vi "Can Expand.vi"(11 "State":T1) -> (3 "Can Expand?":bool)   [LabVIEW 2020, in "Parallel Diagram Block.xnode"]
uses:
  Parallel Diagram Block.xnode
  Parallel Block/Value Type.ctl
  Parallel Block/Parallel Block.lvlib
  Parallel Block/Type Descriptor.ctl
  <vilib>/picture/picture.llb/imagedata.ctl
  Parallel Block/Direction.ctl
  Parallel Block/IO Selection.ctl
  State.ctl
  Parallel Block/Terminal Mode.ctl
  Parallel Block/Terminal Type.ctl
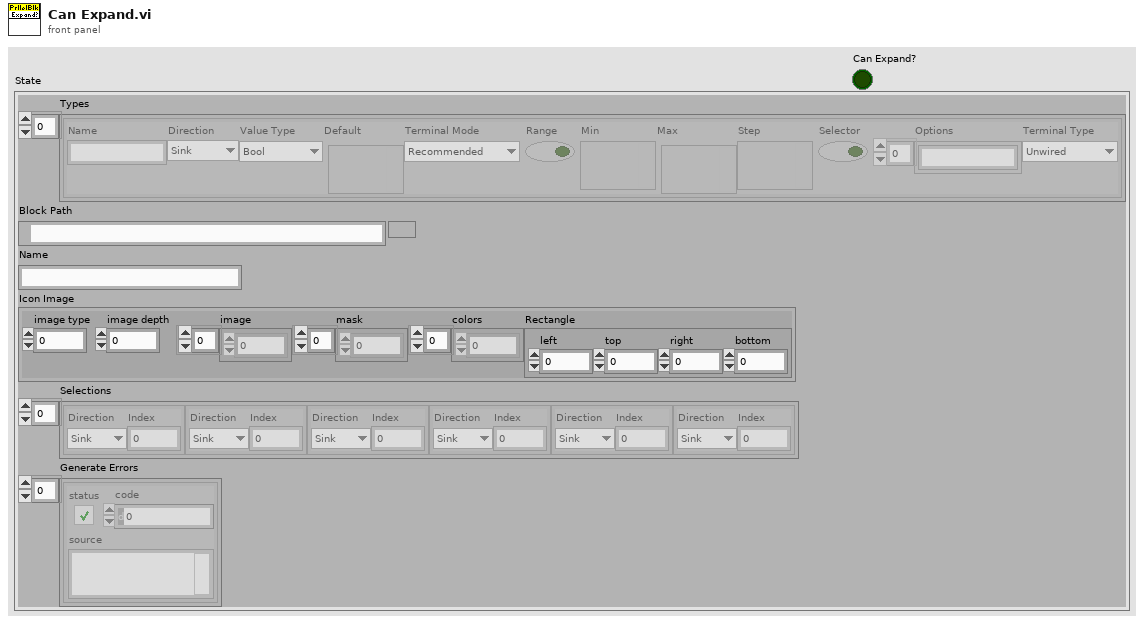
[diagram p1: front panel]
types:
  T1 = typedef "Parallel Diagram Block.xnode/State.ctl" = cluster{"Types":T2[], "Block Path":path, "Name":string, "Icon Image":T7, "Selections":T8[], "Generate Errors":errorcluster[]}
  T2 = typedef "Parallel Block.lvlib/Type Descriptor.ctl" = cluster{"Name":string, "Direction":T3, "Value Type":T4, "Default":variant, "Terminal Mode":T5, "Range":bool, "Min":variant, "Max":variant, "Step":variant, "Selector":bool, "Options":string[], "Terminal Type":T6}
  T3 = typedef "Parallel Block.lvlib/Direction.ctl" = enum16{"Sink", "Source"}
  T4 = typedef "Parallel Block.lvlib/Value Type.ctl" = enum16{"Unknown", "Bool", "U8", "U16", "U32", "U64", "I8", "I16", "I32", "I64", "SGL", "DBL", "CSG", "CDB", "CDBWfm", "String", "DBLWfm"}
  T5 = typedef "Parallel Block.lvlib/Terminal Mode.ctl" = enum16{"Recommended", "Required", "None"}
  T6 = typedef "Parallel Block.lvlib/Terminal Type.ctl" = enum16{"Unwired", "Connection", "Value", "Control Ref"}
  T7 = typedef "imagedata.ctl" = cluster{"image type":i32, "image depth":i32, "image":u8[], "mask":u8[], "colors":u32[], "Rectangle":cluster{"left":i16, "top":i16, "right":i16, "bottom":i16}}
  T8 = typedef "Parallel Block.lvlib/IO Selection.ctl" = cluster{"Direction":T3, "Index":i32}
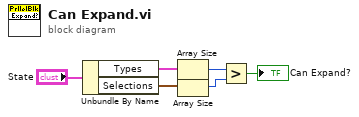
[diagram p0: block diagram]
diagram:
  n1 = Unbundle By Name("State") -> ("Types"=w5:T2[], "Selections"=w4:T8[])
  n2 = Array Size(array=w5) -> (size(s)=w3:i32)
  n3 = Array Size(array=w4) -> (size(s)=w2:i32)
  n4 = Greater?(x=w3, y=w2) -> (0:→"Can Expand?":bool)
